vi "LoadUnloadLimit.vi"(6 "Unload Limit":dbl, 7 "DataFlowIN (Eingang)":T1, 8 "Fehler (Eingang, kein Fehler)":errorcluster, 9 "Load Limit":dbl, 10 "ColHdrString":string[](array[string]), 11 "TableName":string) -> (0 "Fehler (Ausgang)":errorcluster, 1 "DataFlowIN (Ausgang)":T1, 2 "Limit No Car 3":dbl, 3 "Limit No Car 10":dbl)   [LabVIEW 2017]
uses:
  classes/DataCollector.lvclass
  classes/DataHandler.lvclass
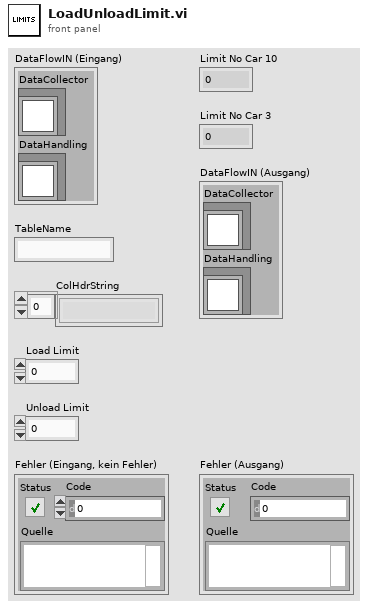
[diagram p1: front panel]
types:
  T1 = cluster{"DataCollector":refnum<class "DataCollector.lvclass">, "DataHandling":refnum<class "DataHandler.lvclass">}
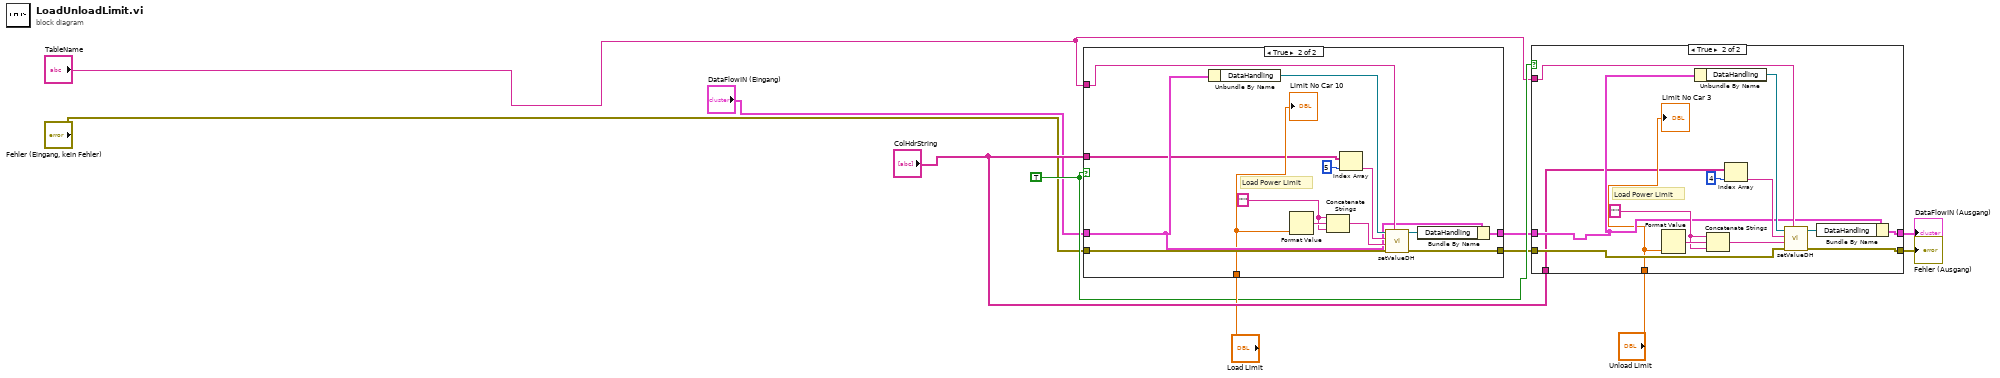
[diagram p0: block diagram]
diagram:
  w8 = TRUE
  n1 = case shown="True" w8 {
    tunnel: [w12 w23] -> w3
    tunnel: [w13 w22] -> w2
    tunnel: "TableName" -> [_ w19]
    tunnel: "Fehler (Eingang, kein Fehler)" -> [w12 w16]
    tunnel: "DataFlowIN (Eingang)" -> [w13 w17]
    tunnel: "Load Limit" -> [_ w15]
    tunnel: "ColHdrString" -> [_ w14]
    frame False {
    }
    frame True {
      w18 = "'" ("String")
      # "Load Power Limit"
      n2 = Unbundle By Name(w17) -> ("DataHandling"=w20:refnum<class "DataHandler.lvclass">)
      n3 = Format Value(value (0)=w15) -> (output string=w25:string)  [unwired: 2 in]
      n4 = Concatenate Strings(w18, w25, w18) -> (w24:string)
      n5 = Index Array(array=w14, index=5) -> (element=w26:string)
      n6 = call-dynamic "setValueDH.vi"("TableName"=w19, "error in (no error)"=w16, "Value"=w24, "ItemName"=w26, "DataHandler in"=w20) -> ("error out"=w23:errorcluster, "DataHandler out"=w21:refnum<class "DataHandler.lvclass">)  [unwired: 5 in]
      n7 = Bundle By Name(cluster=w17, "DataHandling"=w21) -> (w22:T1)
      "Limit No Car 10" <- w15
    }
  }
  n8 = case shown="True" w8 {
    tunnel: [w28 w39] -> w5
    tunnel: [w29 w38] -> w4
    tunnel: "TableName" -> [_ w35]
    tunnel: w3 -> [w28 w32]
    tunnel: w2 -> [w29 w33]
    tunnel: "Unload Limit" -> [_ w31]
    tunnel: "ColHdrString" -> [_ w30]
    frame False {
    }
    frame True {
      w34 = "'" ("String")
      # "Load Power Limit"
      n9 = Format Value(value (0)=w31) -> (output string=w41:string)  [unwired: 2 in]
      n10 = Unbundle By Name(w33) -> ("DataHandling"=w36:refnum<class "DataHandler.lvclass">)
      n11 = Concatenate Strings(w34, w41, w34) -> (w40:string)
      n12 = Index Array(array=w30, index=4) -> (element=w42:string)
      n13 = call-dynamic "setValueDH.vi"("TableName"=w35, "error in (no error)"=w32, "Value"=w40, "ItemName"=w42, "DataHandler in"=w36) -> ("error out"=w39:errorcluster, "DataHandler out"=w37:refnum<class "DataHandler.lvclass">)  [unwired: 5 in]
      n14 = Bundle By Name(cluster=w33, "DataHandling"=w37) -> (w38:T1)
      "Limit No Car 3" <- w31
    }
  }
  "Fehler (Ausgang)" <- w5
  "DataFlowIN (Ausgang)" <- w4
